vi "Calculation_Angle_Between_Displacements-1.vi"(1 "dY 2":dbl, 2 "dX 2":dbl, 3 "dY 1":dbl, 4 "dX 1":dbl) -> (0 "angle in degrees":dbl)   [LabVIEW 2013]
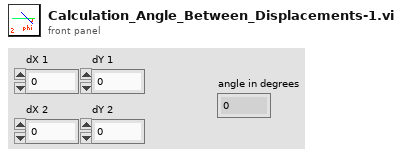
[diagram p1: front panel]
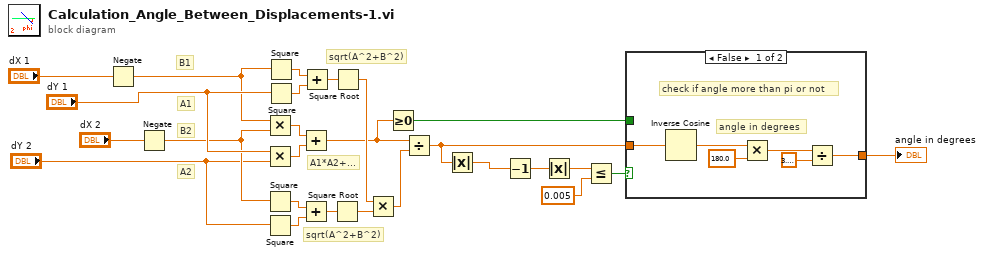
[diagram p0: block diagram]
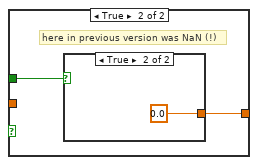
[diagram p2: hidden frame]
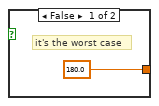
[diagram p3: hidden frame]
diagram:
  # "sqrt(A^2+B^2)"
  # "A1*A2+..."
  # "sqrt(A^2+B^2)"
  # "A2"
  # "B2"
  # "A1"
  # "B1"
  n1 = Negate(x="dX 1") -> (-x=w11:dbl)
  n2 = Negate(x="dX 2") -> (-x=w9:dbl)
  n3 = Multiply(x=w11, y=w9) -> (x*y=w26:dbl)
  n4 = Multiply(x="dY 1", y="dY 2") -> (x*y=w25:dbl)
  n5 = Square(x=w9) -> (x^2=w21:dbl)
  n6 = Square(x="dY 2") -> (x^2=w20:dbl)
  n7 = Square(x=w11) -> (x^2=w24:dbl)
  n8 = Square(x="dY 1") -> (x^2=w23:dbl)
  n9 = Add(x=w26, y=w25) -> (x+y=w15:dbl)
  n10 = Add(x=w21, y=w20) -> (x+y=w19:dbl)
  n11 = Add(x=w24, y=w23) -> (x+y=w22:dbl)
  n12 = Square Root(x=w19) -> (sqrt(x)=w17:dbl)
  n13 = Square Root(x=w22) -> (sqrt(x)=w18:dbl)
  n14 = Multiply(x=w18, y=w17) -> (x*y=w16:dbl)
  n15 = Greater Or Equal To 0?(x=w15) -> (x >= 0?=w14:bool)
  n16 = Divide(x=w15, y=w16) -> (x/y=w3:dbl)
  n17 = Absolute Value(x=w3) -> (abs(x)=w2:dbl)
  n18 = Decrement(x=w2) -> (x-1=w1:dbl)
  n19 = Absolute Value(x=w1) -> (abs(x)=w6:dbl)
  n20 = Less Or Equal?(x=w6, y=0.005) -> (x <= y?=w4:bool)
  n21 = case shown="False" w4 {
    tunnel: w14 -> [_ w33]
    tunnel: [w29 w34] -> w7
    tunnel: w3 -> [w28 _]
    frame False {
      # "check if angle more than pi or not"
      # "angle in degrees"
      n22 = Inverse Cosine(1:w28) -> (0:w27:dbl)
      n23 = Multiply(x=w27, y=180.0) -> (x*y=w31:dbl)
      n24 = Divide(x=w31, y=3.141592653589793) -> (x/y=w29:dbl)
    }
    frame True {
      # "here in previous version was NaN (!)"
      n25 = case shown="True" w33 {
        tunnel: [180.0 0.0] -> w34
        frame False {
          # "it's the worst case"
        }
        frame True {
        }
      }
    }
  }
  "angle in degrees" <- w7
